vi "Lvi Get Error String.vi"(11 "err":i32) -> (2 "function return":string, 3 "StringLength":i32)   [LabVIEW 2016, in "DtLvLink.lvlib"]
doc: "Calls directly into the entry points of the DLL of the Data Acq SDK to return the description of the error. This VI is used by the higher-level VI, DtOLErrorParser."
uses:
  <userlib>/LV-Link3/DtLvLink.lvlib
  <userlib>/LV-Link3/DtLvLink_32.dll
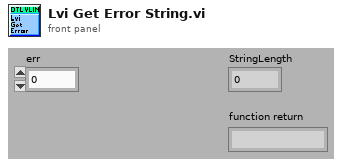
[diagram p1: front panel]
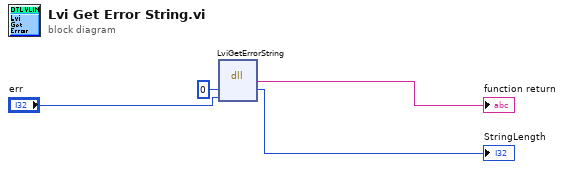
[diagram p0: block diagram]
diagram:
  n1 = dll-call lib="C:/Program Files (x86)/National Instruments/LabVIEW 2016/user.lib/LV-Link3/DtLvLink_32.*" fn="LviGetErrorString"("StringLength"=0, "err"="err") -> (→"function return":string, "StringLength"=→"StringLength":i32)  [unwired: 4 in, 2 out]
